vi "Area_Scan_v12 (SubVI).vi"(0 "Step Axis":string="2", 1 "Scan Termination":T1(ring)=enum."End Position", 2 "Center of Scan":bool=TRUE, 3 "Scan Type":enum16{"Sinusoidal", "Spiral"}(ring), 4 "Analog Input":i32=1, 5 "Table rate":i32=5, 6 "System no.":i32, 7 "error in (no error)":errorcluster, 8 "Mesh in":dbl=0.1, 9 "X-frequency":dbl=2.0, 10 "X Scan Range":dbl=10.0, 11 "Y-velocity":dbl=2.0, 12 "Y Scan Range":dbl=10.0, 14 "X Scan Center":dbl, 16 "Y Scan Center":dbl) -> (18 "3D Line Graph":refnum<class "Base Datatype.lvclass">[](array[class]), 20 "Intensity Graph":dbl[][](array[numeric]), 25 "Nano AS Data":dbl[][](array[numeric]), 26 "AS Duration (msec)":u32, 27 "error out":errorcluster)   [LabVIEW 2023]
uses:
  <vilib>/Native 3D Graph/classes/Base Datatype.lvclass
  <vilib>/Native 3D Graph/xcontrol/3DPC_SurfacePlot.xctl
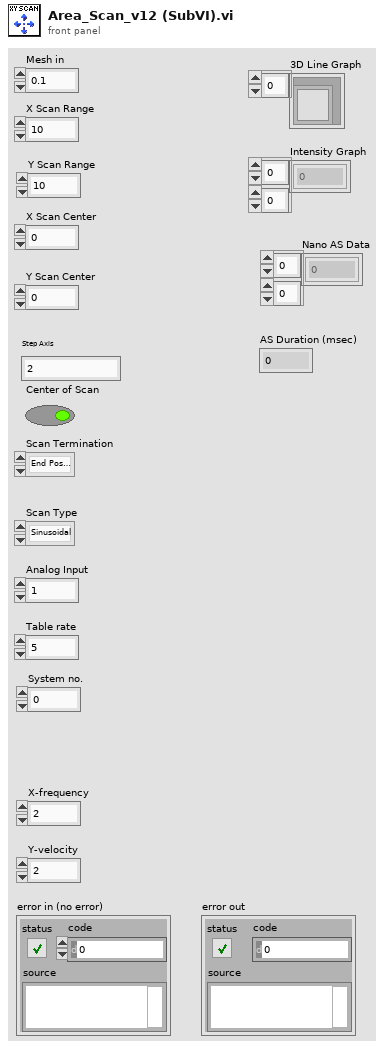
[diagram p1: front panel]
types:
  T1 = enum16{"Maximum", "End Position", "Center of scan", ""}
  T2 = cluster{"Set target type?":bool, "Target type":i32}
  T3 = cluster{"Set stop pos. option?":bool, "Stop pos. option":i32}
  T4 = cluster{"Set centroid method?":bool, "Centroid method":i32}
  T5 = cluster{"Step axis":string, "Range step axis":dbl, "Set Mid. pos?":bool, "Mid. pos. step axis":dbl}
  T6 = cluster{"Scan axis":string, "Range scan axis":dbl, "Set Mid. pos?":bool, "Mid. pos. scan axis":dbl}
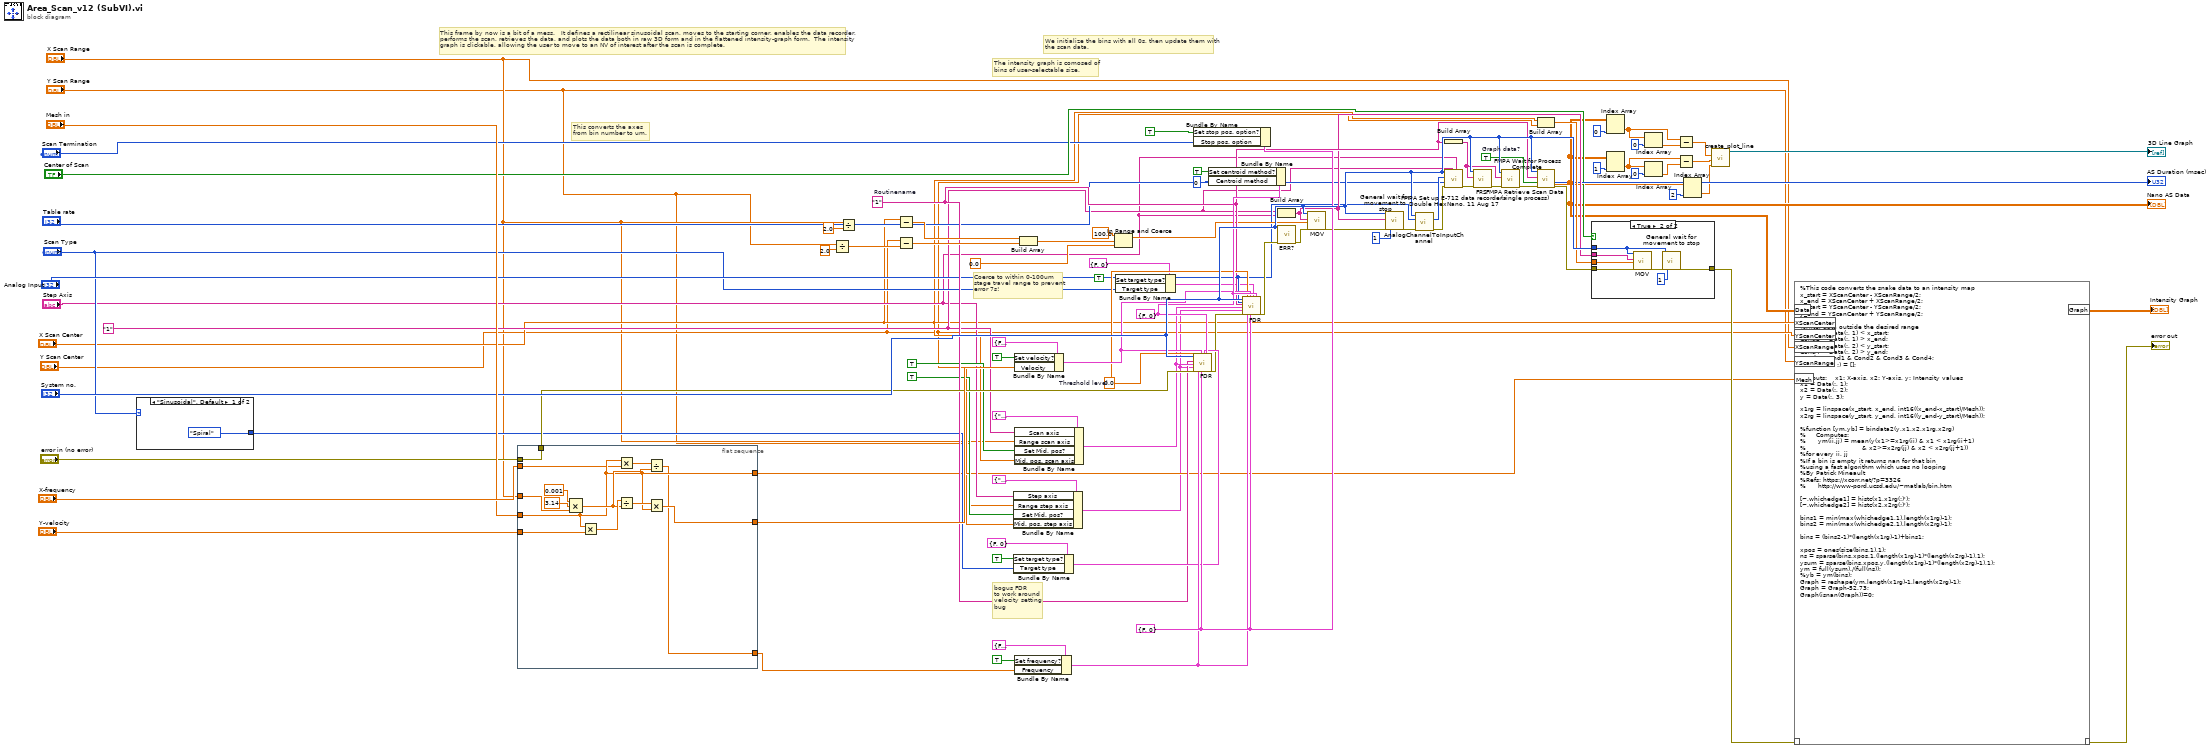
[diagram p0: block diagram]
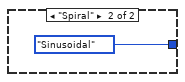
[diagram p2: hidden frame]
diagram:
  w13 = "1"
  w45 = TRUE  # Graph data?
  w77 = T3 {"Set stop pos. option?"=FALSE, "Stop pos. option"=0} ("Stop position option settings")
  w75 = T4 {"Set centroid method?"=FALSE, "Centroid method"=0} ("Centroid method settings")
  w73 = 0.0  # Threshold level
  w68 = "1"  # Routinename
  # "This converts the axes\nfrom bin number to um."
  # "We initialize the bins with all 0s, then update them with\nthe scan data."
  # "The intensity graph is comosed of\nbins of user-selectable size."
  # "This frame by now is a bit of a mess.   It defines a rectilinear sinusoidal scan, moves to the starting corner, enables the data recorder,\nperforms the scan, retrieves the data, and plots the data both in raw 3D form and in the flattened intensity-graph form.  The intensity\ngraph is clickable, allowing the user to move to an NV of interest after the scan is complete."
  # "bogus FDR\nto work around\nvelocity setting\nbug"
  # "Coerce to within 0-100um\nstage travel range to prevent\nerror 7s!"
  n1 = case shown="\"Sinusoidal\", Default" "Scan Type" {
    tunnel: [enum16{"Sinusoidal", "Spiral"}."Spiral" ("Scan Type") enum16{"Sinusoidal", "Spiral"}."Sinusoidal" ("Scan Type")] -> w17
    frame "Sinusoidal", Default {
    }
    frame "Spiral" {
    }
  }
  n2 = flat-sequence {
    tunnel: "X Scan Range" -> [w102]
    tunnel: [w98] -> w82
    tunnel: "error in (no error)" -> [w98]
    tunnel: "Mesh in" -> [w97]
    tunnel: "X-frequency" -> [w96]
    tunnel: "Y-velocity" -> [w95]
    tunnel: [w97] -> w6
    tunnel: [w94] -> w90
    tunnel: [w93] -> w89
    frame #0 {
      n3 = Compound Arithmetic op=MULTIPLY(0.001, 3.14, w102) -> (w100:dbl)
      n4 = Multiply(x=w97, y=w95) -> (x*y=w101:dbl)
      n5 = Multiply(x=w97, y=w96) -> (x*y=w105:dbl)
      n6 = Divide(x=w101, y=w100) -> (x/y=w99:dbl)
      n7 = Divide(x=w105, y=w100) -> (x/y=w93:dbl)
      n8 = Multiply(x=w99, y=w97) -> (x*y=w94:dbl)
    }
  }
  n9 = Divide(x="Y Scan Range", y=2.0) -> (x/y=w66:dbl)
  n10 = Divide(x="X Scan Range", y=2.0) -> (x/y=w33:dbl)
  n11 = Subtract(x="X Scan Center", y=w33) -> (x-y=w85:dbl)
  n12 = Subtract(x="Y Scan Center", y=w66) -> (x-y=w86:dbl)
  n13 = Bundle By Name(cluster=T5 {"Step axis"="", "Range step axis"=0.1, "Set Mid. pos?"=FALSE, "Mid. pos. step axis"=0.1} ("Step axis settings"), "Step axis"="Step Axis", "Range step axis"="Y Scan Range", "Set Mid. pos?"=TRUE, "Mid. pos. step axis"="Y Scan Center") -> (w1:T5)
  n14 = Bundle By Name(cluster=T2 {"Set target type?"=FALSE, "Target type"=0} ("Target type settings"), "Set target type?"=TRUE, "Target type"=w17) -> (w72:T2)
  n15 = Bundle By Name(cluster=cluster{"Set velocity?":bool, "Velocity":dbl} {"Set velocity?"=FALSE, "Velocity"=0.1} ("Velocity settings"), "Set velocity?"=TRUE ("Set target type?"), "Velocity"=w90) -> (w74:cluster{"Set velocity?":bool, "Velocity":dbl})
  n16 = Bundle By Name(cluster=T6 {"Scan axis"="", "Range scan axis"=0.1, "Set Mid. pos?"=FALSE, "Mid. pos. scan axis"=0.1} ("Scan axis settings"), "Scan axis"=w13, "Range scan axis"="X Scan Range", "Set Mid. pos?"=TRUE, "Mid. pos. scan axis"="X Scan Center") -> (w69:T6)
  n17 = Bundle By Name(cluster=cluster{"Set frequency?":bool, "Frequency":dbl} {"Set frequency?"=FALSE, "Frequency"=10.0} ("Frequency settings"), "Set frequency?"=TRUE, "Frequency"=w89) -> (w76:cluster{"Set frequency?":bool, "Frequency":dbl})
  n18 = Build Array(w85, w86) -> (w64:dbl[])
  n19 = In Range and Coerce(upper limit=100.0, x=w64, lower limit=0.0) -> (coerced(x)=w65:dbl[])  [unwired: 1 out]
  n20 = Bundle By Name(cluster=T2 {"Set target type?"=FALSE, "Target type"=0} ("Target type settings"), "Set target type?"=TRUE, "Target type"="Scan Type") -> (w24:T2)
  n21 = Bundle By Name(cluster=w77, "Set stop pos. option?"=TRUE, "Stop pos. option"="Scan Termination") -> ()  [unwired: 1 out]
  n22 = call "FDR.vi"("System no."="System no.", "Routinename"=w68, "Scan axis settings"=w69, "Step axis settings"=w1, "error in"=w82, "Threshold level"=w73, "Frequency settings"=w76, "Velocity settings"=w74, "Stop position option settings"=w77, "Target type settings"=w72, "Centroid method settings"=w75) -> ("error out"=w67:errorcluster)  [unwired: 3 in, 5 out]
  n23 = Bundle By Name(cluster=w75, "Set centroid method?"=TRUE, "Centroid method"=0) -> ()  [unwired: 1 out]
  n24 = call "FDR.vi"("System no."="System no.", "Board"="Analog Input", "Routinename"=w68, "Scan axis settings"=w69, "Step axis settings"=w1, "error in"=w67, "Threshold level"=w73, "Frequency settings"=w76, "Velocity settings"=w74, "Stop position option settings"=w77, "Target type settings"=w24, "Centroid method settings"=w75) -> ("error out"=w51:errorcluster)  [unwired: 2 in, 5 out]
  n25 = Build Array(w13, "Step Axis") -> (w48:string[])
  n26 = call "ERR?.vi"("System no."="System no.", "error in"=w51) -> ("error out"=w52:errorcluster)  [unwired: 16 in, 1 out]
  n27 = call "MOV.vi"("System no."="System no.", "Axes to move"=w48, "Position values"=w65, "error in"=w52) -> ("error out"=w35:errorcluster)  [unwired: 1 in, 14 out]
  n28 = call "General wait for movement to stop.vi"("System no."="System no.", "Axes to wait for"=w48, "error in"=w35, "Polling cycle \ntime, ms"=u32 1 ("Polling cycle \ntime, ms")) -> ("error out"=w36:errorcluster)  [unwired: 4 in, 11 out]
  n29 = call "AnalogChannelToInputChannel.vi"("error in (no error)"=w36, "Optical Channel In"="Analog Input", "System no."="System no.") -> ("error out"=w39:errorcluster, "Input Channel Out"=w46:i32)  [unwired: 7 in]
  n30 = Build Array(w68) -> (w44:string[])
  n31 = call "FMPA Set up E-712 data recorder - Double HexNano, 11 Aug 17.vi"("Step axis sensor ch"="Step Axis", "Scan axis sensor ch"=w13, "error in"=w39, "Table rate"="Table rate", "Opt. Ch."=w46, "System no."="System no.") -> ("error out"=w41:errorcluster)  [unwired: 5 in]
  n32 = call "FRS.vi"("System no."="System no.", "Routines to start"=w44, "error in"=w41) -> ("error out"=w42:errorcluster)  [unwired: 16 in]
  n33 = call "FMPA Wait for Process Complete.vi"("error in"=w42, "Routines to query"=w44, "System no."="System no.") -> ("error out"=w43:errorcluster)  [unwired: 7 in, 1 out]
  n34 = Build Array("X Scan Center", "Y Scan Center") -> (w47:dbl[])
  n35 = call "FMPA Retrieve Scan Data (single process).vi"("System no."="System no.", "Process"=w68, "Graph data?"=w45, "error in"=w43) -> ("Duration (msec)"=→"AS Duration (msec)":u32, "Data"=w10:dbl[][], "error out"=w49:errorcluster)  [unwired: 10 in, 3 out]
  "Nano AS Data" <- w10
  n36 = case shown="True" "Center of Scan" {
    tunnel: w47 -> [_ w111]
    tunnel: w48 -> [_ w110]
    tunnel: w49 -> [w106 w109]
    tunnel: "System no." -> [_ w108]
    tunnel: [w106 w107] -> w9
    frame False {
    }
    frame True {
      n37 = call "MOV.vi"("System no."=w108, "Axes to move"=w110, "Position values"=w111, "error in"=w109) -> ("error out"=w113:errorcluster)  [unwired: 1 in, 14 out]
      n38 = call "General wait for movement to stop.vi"("System no."=w108, "error in"=w113, "Polling cycle \ntime, ms"=u32 1 ("Polling cycle \ntime, ms")) -> ("error out"=w107:errorcluster)  [unwired: 5 in, 11 out]
    }
  }
  n39 = Index Array(array=w10, index (col)=0 ("index")) -> (element=w56:dbl[])  [unwired: 1 in]
  n40 = Index Array(array=w10, index (col)=1 ("index")) -> (element=w53:dbl[])  [unwired: 1 in]
  n41 = Index Array(array=w56, index=0) -> (element=w57:dbl)
  n42 = Index Array(array=w53, index=0) -> (element=w54:dbl)
  n43 = Subtract(x=w56, y=w57) -> (x-y=w79:dbl[])
  n44 = Subtract(x=w53, y=w54) -> (x-y=w80:dbl[])
  n45 = Index Array(array=w10, index (col)=2 ("index")) -> (element=w11:dbl[])  [unwired: 1 in]
  n46 = call <vilib>:"create_plot_line.vi"("z vector"=w11, "y vector"=w80, "x vector"=w79) -> ("plots out"=→"3D Line Graph":refnum<class "Base Datatype.lvclass">[])  [unwired: 2 in, 6 out]
  n47 = script code="%This code converts the snake data to an intensity map\nx_start = XScanCenter - XScanRange/2;\nx_end = XScanCenter + XScanRange/2;\ny_start = YScanCenter - YScanRange/2;\ny_end = YScanCenter + YScanRange/2;\n\n%Filter data outside the desired range\nCond1 = Data(:, 1) < x_start;\nCond2 = Data(:, 1) > x_end;\nCond3 = Data(:, 2) < y_start;\nCond4 = Data(:, 2) > y_end;\nCond = Cond1 & Cond2 & Cond3 & Cond4;\nData(Cond, :) = [];\n\n%Inputs:    x1: X-axis, x2: Y-axis, y: Intensity values\nx1 = Data(:, 1);\nx2 = Data(:, 2);\ny = Data(:, 3);\n\nx1rg = linspace(x_start, x_end, int16((x_end-x_start)/Mesh));\nx2rg = linspace(y_start, y_end, int16((y_end-y_start)/Mesh));\n\n%function [ym,yb] = bindata2(y,x1,x2,x1rg,x2rg)\n%     Computes:\n%      ym(ii,jj) = mean(y(x1>=x1rg(ii) & x1 < x1rg(ii+1) \n%                            & x2>=x2rg(jj) & x2 < x2rg(jj+1))\n%for every ii, jj\n%If a bin is empty it returns nan for that bin\n%using a fast algorithm which uses no looping\n%By Patrick Mineault\n%Refs: https://xcorr.net/?p=3326\n%      http://www-pord.ucsd.edu/~matlab/bin.htm\n\n[~,whichedge1] = histc(x1,x1rg(:)');\n[~,whichedge2] = histc(x2,x2rg(:)');\n\nbins1 = min(max(whichedge1,1),length(x1rg)-1);\nbins2 = min(max(whichedge2,1),length(x2rg)-1);\n\nbins = (bins2-1)*(length(x1rg)-1)+bins1;\n\nxpos = ones(size(bins,1),1);\nns = sparse(bins,xpos,1,(length(x1rg)-1)*(length(x2rg)-1),1);\nysum = sparse(bins,xpos,y,(length(x1rg)-1)*(length(x2rg)-1),1);\nym = full(ysum)./(full(ns));\n%yb = ym(bins);\nGraph = reshape(ym,length(x1rg)-1,length(x2rg)-1);\nGraph = Graph-52.73;\nGraph(isnan(Graph))=0;"("??"=w9, "Data"=w10, "Mesh"=w6, "XScanCenter"="X Scan Center", "YScanCenter"="Y Scan Center", "XScanRange"="X Scan Range", "YScanRange"="Y Scan Range") -> ("??"=→"error out":errorcluster, "Graph"=→"Intensity Graph":dbl[][])
